vi "TCP Write Alive 2.vi"(0 "remote port or service name":u16=6341, 1 "MultiCast Port":u16=58432, 3 "Stopqueue":refnum<queue>, 5 "address":string="localhost", 7 "Stop":bool, 9 "Name":string="MyName 2", 11 "error in (no error)":errorcluster, 13 "MultiCast Address":string="234.5.6.7", 14 "stop":bool) -> (4 "Stop?":bool, 6 "PhysicalStop?":bool, 15 "error out":errorcluster)   [LabVIEW 2013]
uses:
  <vilib>/Utility/tcp.llb/UDP Multicast Read-Only Open.vi
panel:
  out "stop 2":bool
  in  "OK":bool
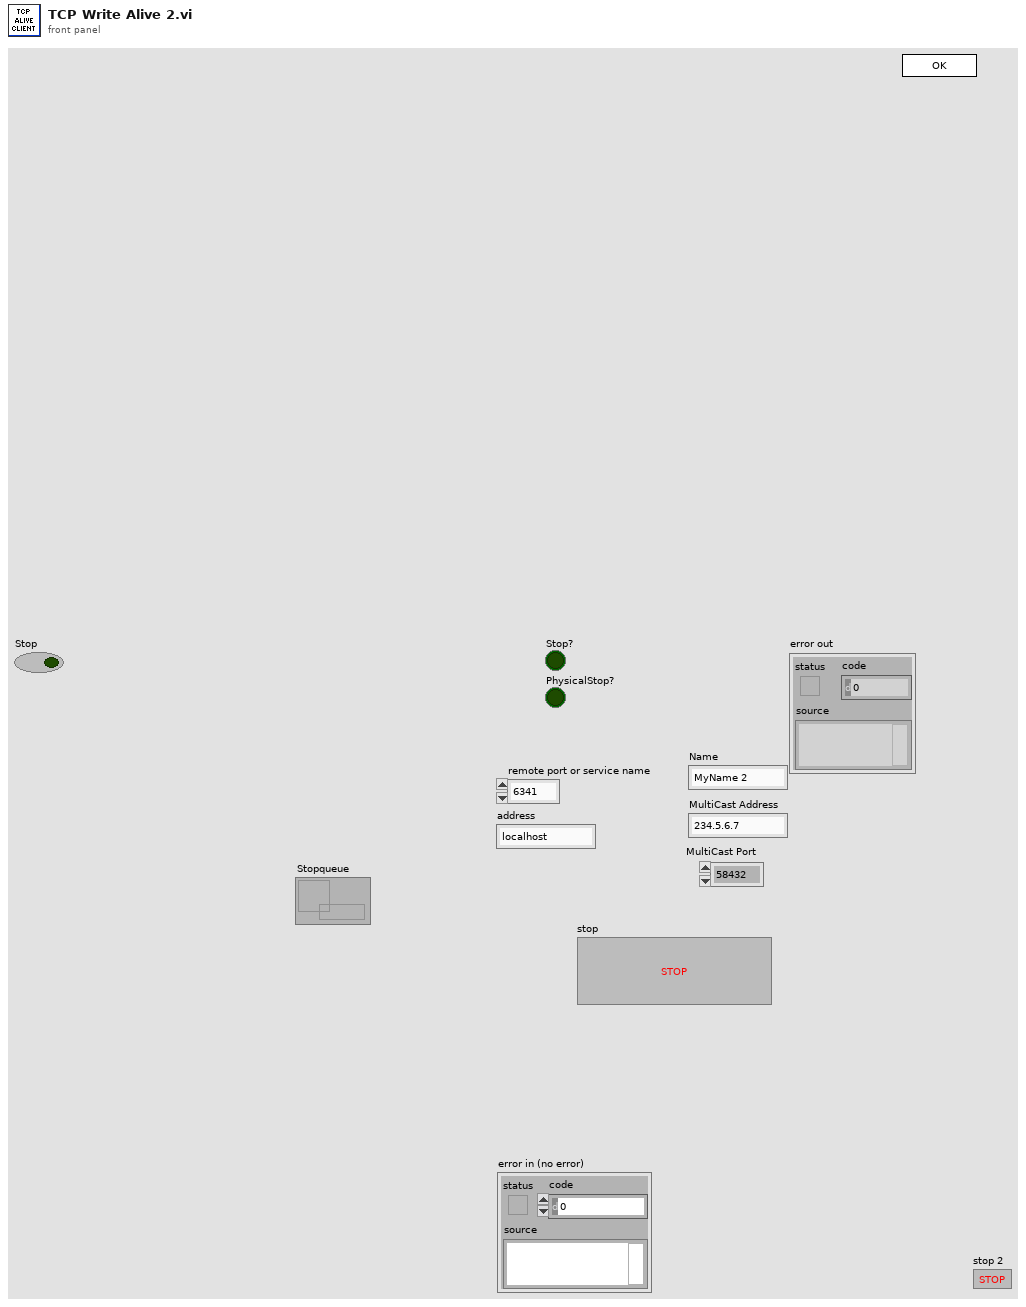
[diagram p1: front panel]
types:
  T1 = enum32{"invalid app kind", "Development System", "Run Time System", "Student Edition", "Embedded LabVIEW", "Evaluation", "Custom"}
  T2 = enum32{"Invalid", "Standard", "Closed", "Hidden", "Minimized", "Maximized"}
  T3 = cluster{"Core":cluster{"Current VI Reference":refnum<vi>, "Close Panel on Exit?":bool}, "PhysicalStop?":bool, "Alive String":string, "connection ID":refnum<k5>, "Address":string, "remote port or service name 2":u16, "Stop String":string}
  T4 = cluster{"Current VI Reference":refnum<vi>, "Close Panel on Exit?":bool}
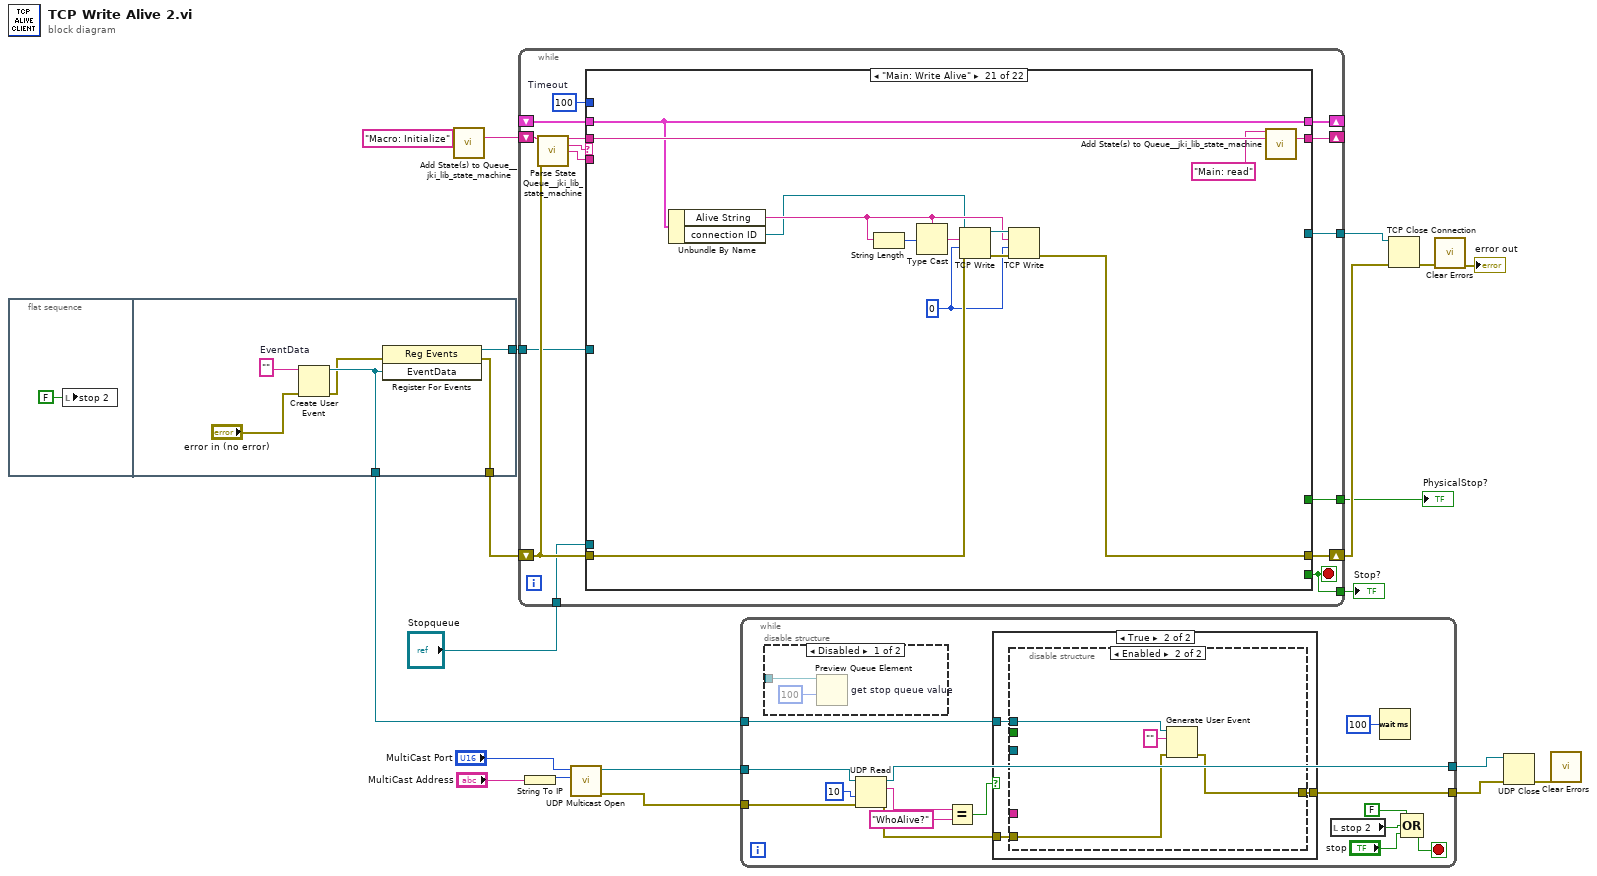
[diagram p0: block diagram]
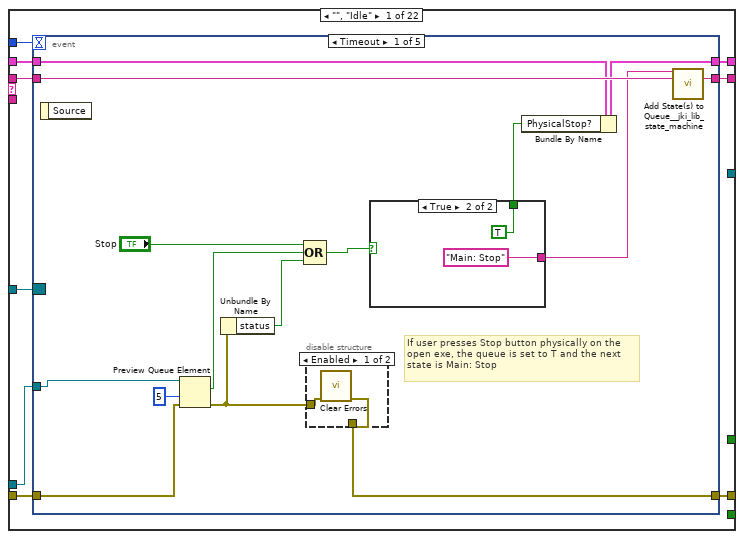
[diagram p2: hidden frame]
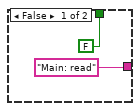
[diagram p4: hidden frame]
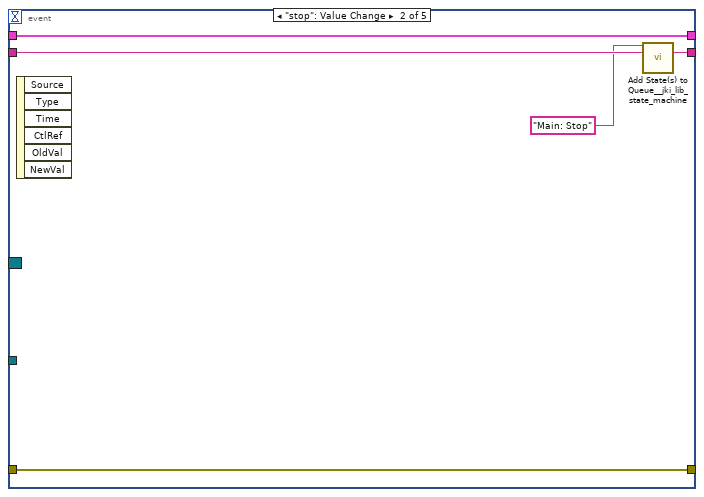
[diagram p5: hidden frame]
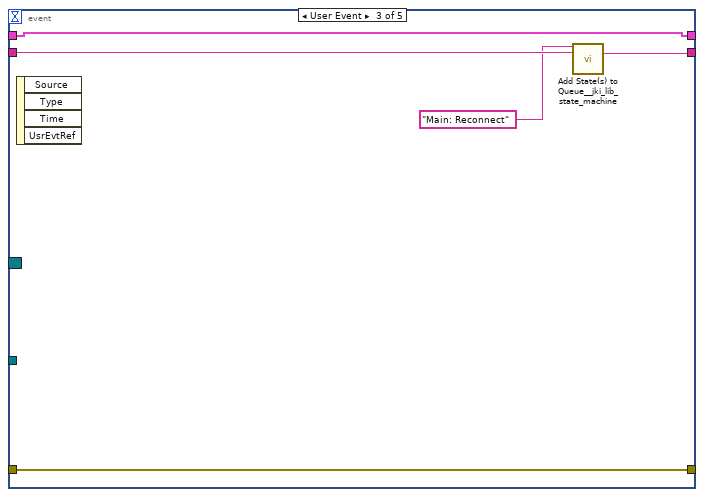
[diagram p6: hidden frame]
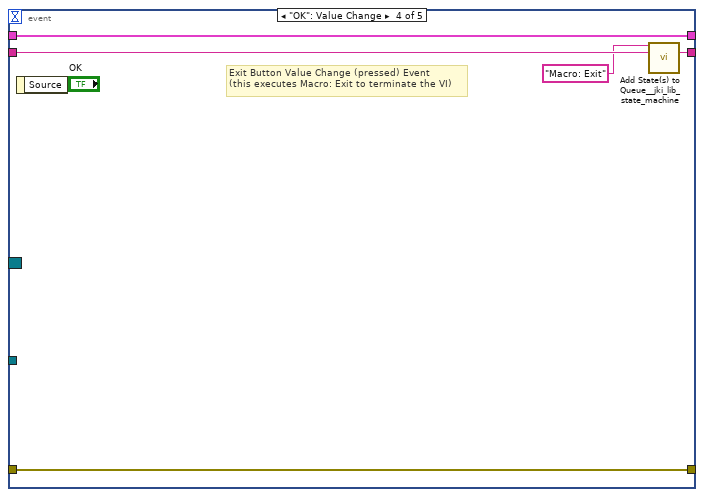
[diagram p7: hidden frame]
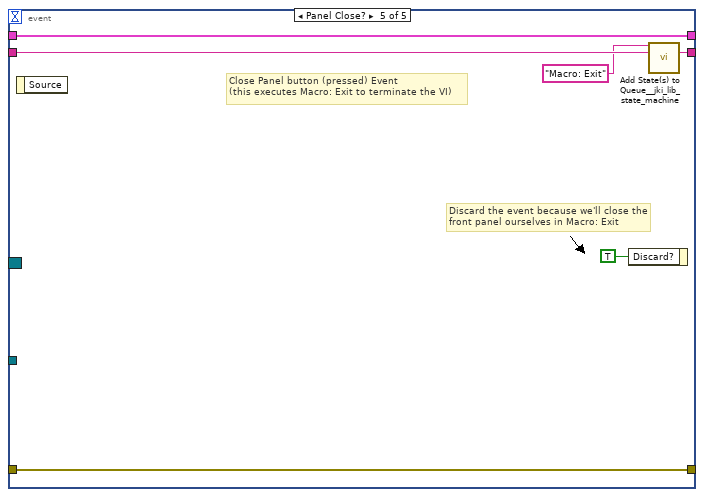
[diagram p8: hidden frame]
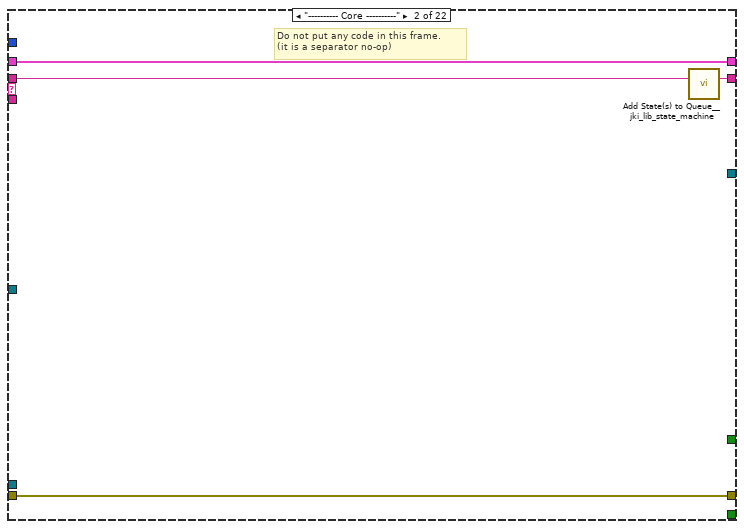
[diagram p9: hidden frame]
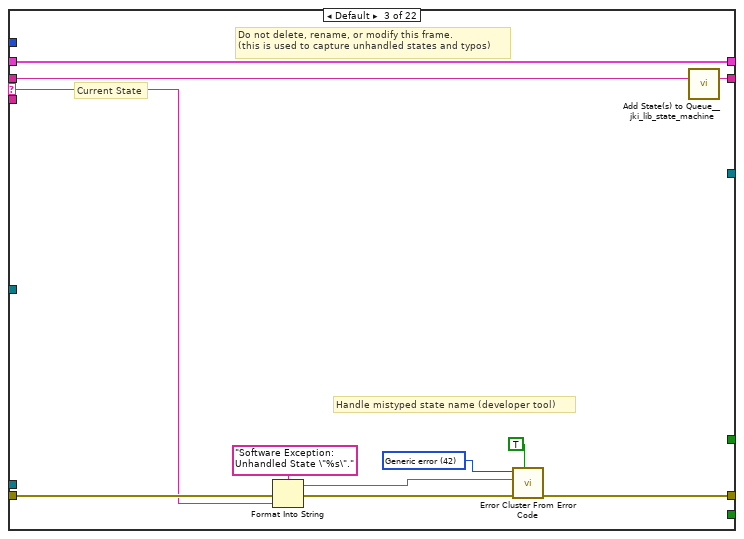
[diagram p10: hidden frame]
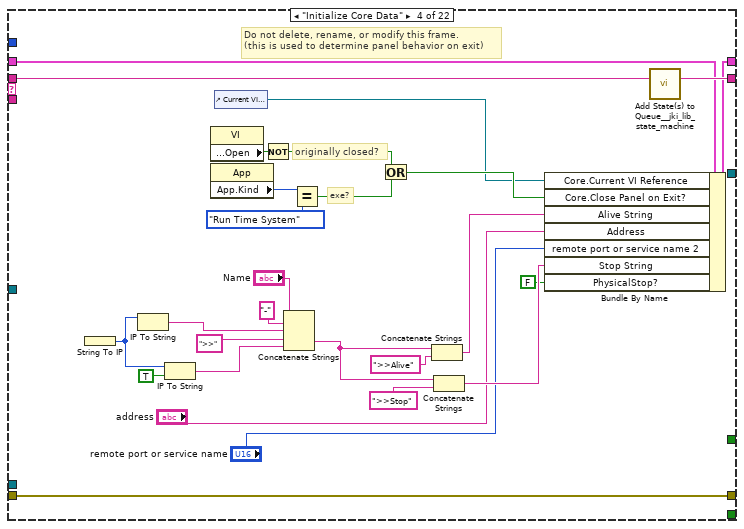
[diagram p11: hidden frame]
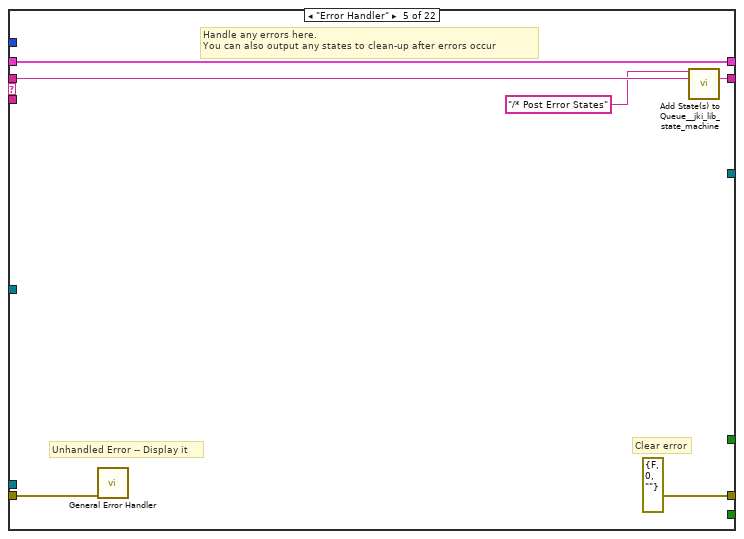
[diagram p12: hidden frame]
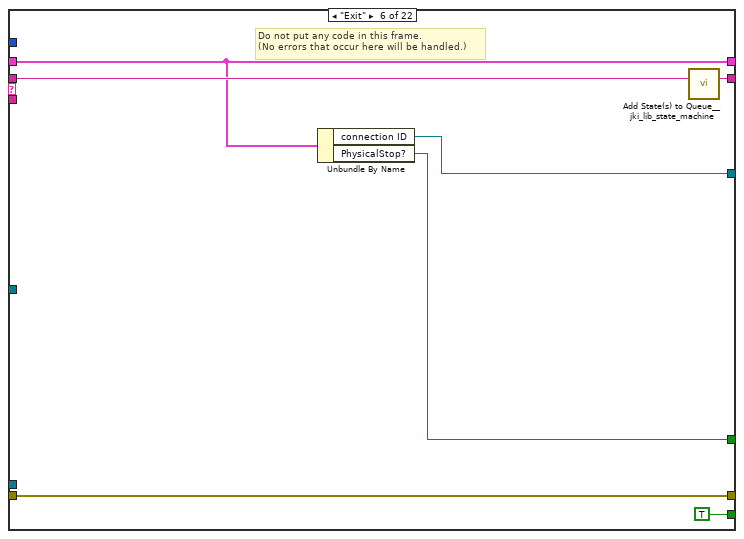
[diagram p13: hidden frame]
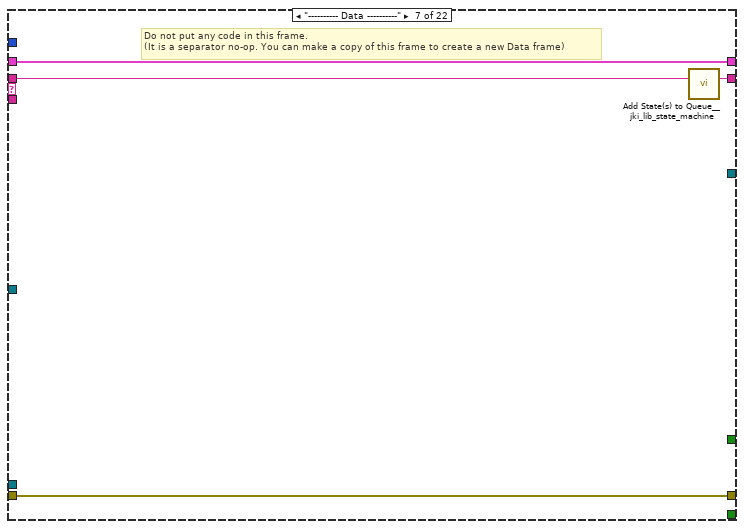
[diagram p14: hidden frame]
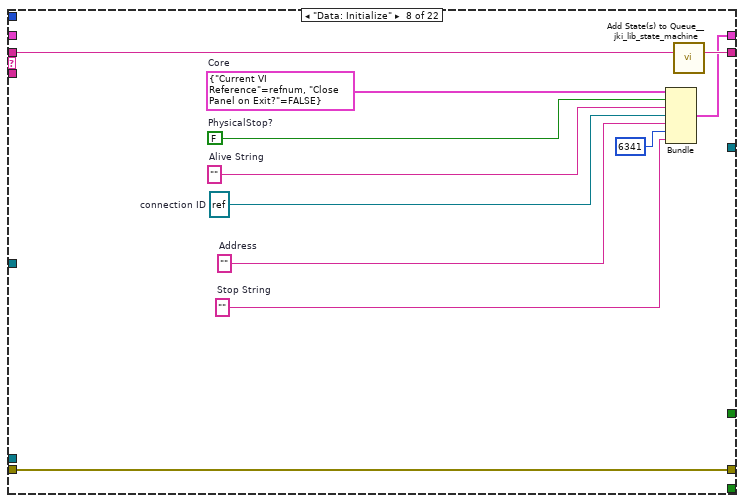
[diagram p15: hidden frame]
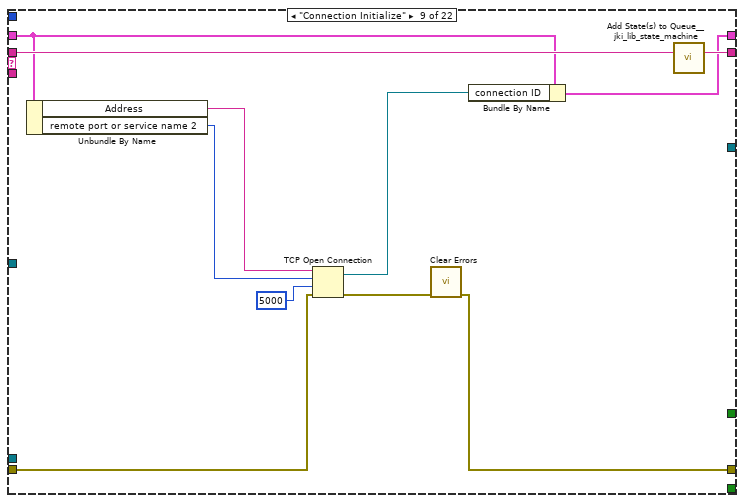
[diagram p16: hidden frame]
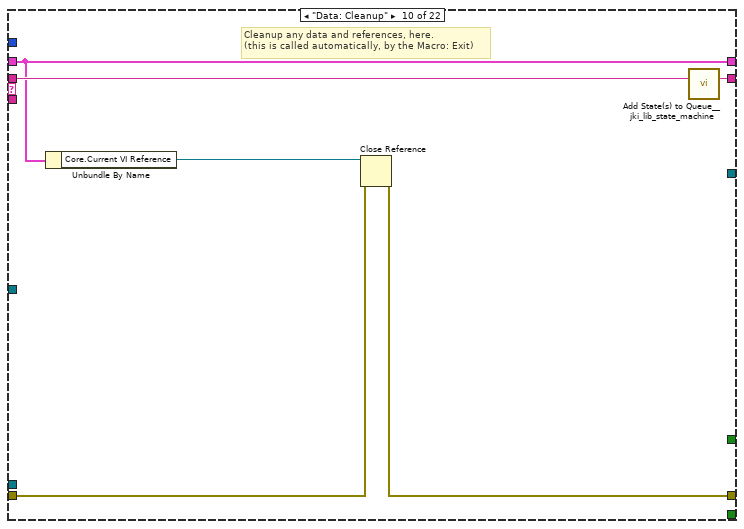
[diagram p17: hidden frame]
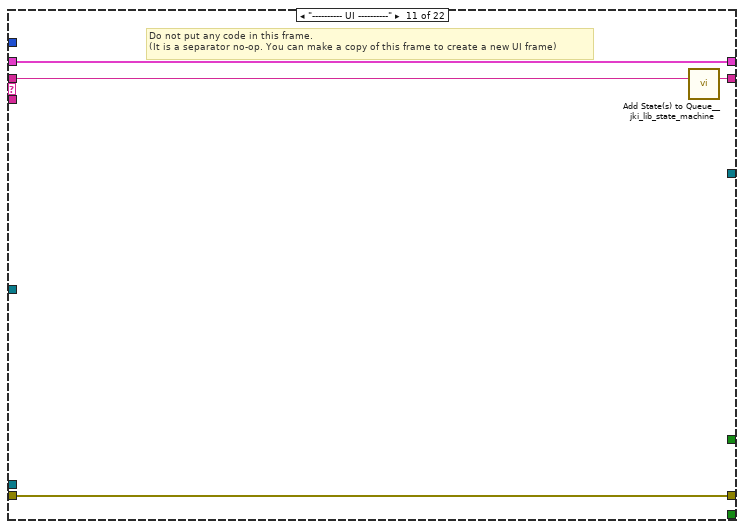
[diagram p18: hidden frame]
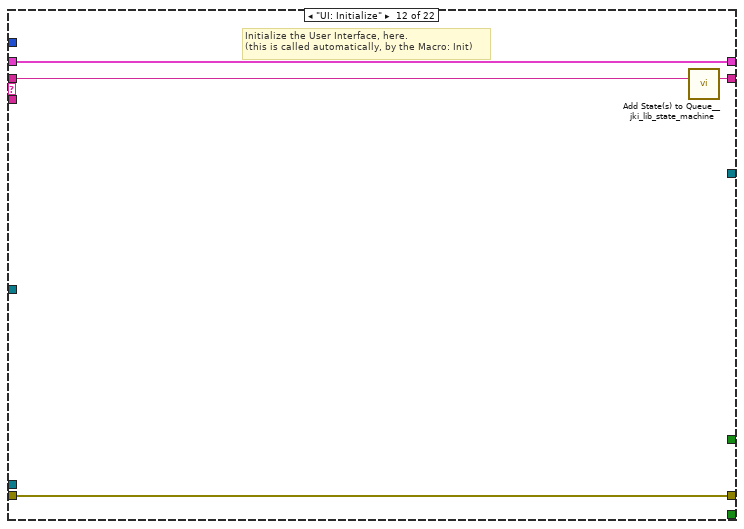
[diagram p19: hidden frame]
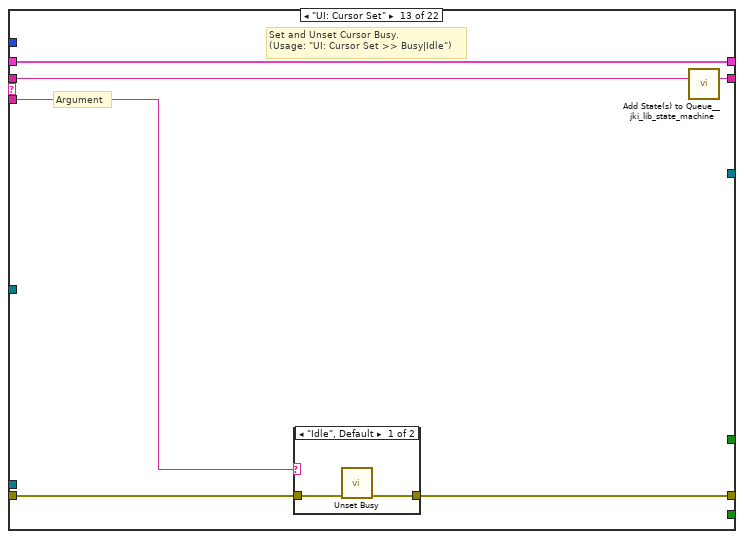
[diagram p20: hidden frame]
diagram:
  n1 = flat-sequence {
    tunnel: [w27] -> w11
    tunnel: [w25] -> w10
    tunnel: [w22] -> w9
    frame #0 {
      n2 = local write "stop 2"(FALSE ("stop 2")) -> ()
    }
    frame #1 {
      w26 = ""  # EventData
      n3 = Create User Event(user event datatype=w26, error in="error in (no error)") -> (user event=w25:refnum<user-event>, error out=w23:errorcluster)
      n4 = register-events(error in=w23, w25) -> (reference out=w27:refnum<event-registration>, error out=w22:errorcluster)  [unwired: 1 in]
    }
  }
  n5 = call <vilib>:"Add State(s) to Queue__jki_lib_state_machine.vi"("State(s) in (\"\")"="Macro: Initialize") -> ("States Out"=w13:string)  [unwired: 14 in]
  n6 = while {
    shift-right: [w36] -> _
    shift-left: _ -> [w35]
    shift-right: [w38] -> w6
    shift-left: w9 -> [w33]
    shift-right: [w37] -> _
    shift-left: w13 -> [w39]
    tunnel: w11 -> [w32]
    tunnel: [w31] -> w7
    tunnel: "Stopqueue" -> [w30]
    tunnel: [w29] -> w3
    tunnel: [w28] -> w1
    stop <- w29 stop-if-true
    w34 = 100  # Timeout
    n7 = call <vilib>:"Parse State Queue__jki_lib_state_machine.vi"("State Queue"=w39, "Error In (no error)"=w33) -> ("Remaining States"=w41:string, "Current State"=w42:string, "Arguments"=w40:string)  [unwired: 11 in]
    n8 = case shown="\"Main: Write Alive\"" w42 {
      selector: w42 -> [_ _ w99 _ _ _ _ _ _ _ _ _ _ _ _ _ _ _ _ _ _ _]
      tunnel: w41 -> [w51 w98 w103 w136 w142 w149 w153 w164 w175 w181 w185 w189 w195 w206 w232 w237 w247 w251 w266 w290 w322 w340]
      tunnel: w40 -> [_ _ _ _ _ _ _ _ _ _ _ _ w190 w200 _ _ _ _ _ _ _ _]
      tunnel: w35 -> [w49 w95 w101 w127 w139 w145 w150 _ w171 w176 w182 w187 w193 w202 w229 w234 w244 w248 w262 w273 w316 w334]
      tunnel: [w48 w96 w105 w133 errorcluster {"status"=FALSE, "code"=0, "source"=""} ("error out") w147 w151 w161 w166 w177 w183 w186 w191 w203 w230 w235 w245 w249 w254 w276 w310 w326] -> w38
      tunnel: w33 -> [w47 w96 w104 w133 w138 w147 w151 w161 w167 w178 w183 w186 w192 w204 w230 w235 w245 w249 w254 w277 w313 w331]
      tunnel: [w50 w97 w102 w135 w141 w148 w152 w163 w174 w180 w184 w188 w194 w205 w231 w236 w246 w250 w265 w289 w321 w339] -> w37
      tunnel: [_ _ _ _ _ TRUE _ _ _ _ _ _ _ _ _ _ _ _ _ _ _ _] -> w29
      tunnel: [w46 w95 w101 w134 w139 w145 w150 w162 w173 w176 w182 w187 w193 w202 w229 w234 w244 w248 w261 w272 w316 w334] -> w36
      tunnel: w34 -> [w45 _ _ _ _ _ _ _ _ _ _ _ _ _ _ _ _ _ _ _ _ _]
      tunnel: w32 -> [w44 _ _ _ _ _ _ _ _ _ _ _ _ _ _ _ _ _ _ _ _ _]
      tunnel: [_ _ _ _ _ w144 _ _ _ _ _ _ _ _ _ _ _ _ _ _ _ _] -> w31
      tunnel: w30 -> [w43 _ _ _ _ _ _ _ _ _ _ _ _ _ _ _ _ _ _ _ _ w325]
      tunnel: [_ _ _ _ _ w143 _ _ _ _ _ _ _ _ _ _ _ _ _ _ _ _] -> w28
      frame "", "Idle" {
        n9 = event shown="[0] Timeout" {
          selector: w44 -> [_ _ _ _ _]
          dyn-events: _ -> [_ _ _ _ _]
          timeout: w45 -> [_ _ _ _ _]
          tunnel: w51 -> [w66 w77 w82 w88 w94]
          tunnel: [w65 w78 w83 w87 w93] -> w50
          tunnel: w49 -> [w61 w76 w80 w85 w91]
          tunnel: [w57 w74 w79 w86 w92] -> w48
          tunnel: w47 -> [w58 w74 w79 w86 w92]
          tunnel: [w60 w76 w80 w85 w91] -> w46
          tunnel: w43 -> [w63 _ _ _ _]
          event Timeout {
            # "If user presses Stop button physically on the\nopen exe, the queue is set to T and the next\nstate is Main: Stop"
            n10 = event-data() -> ()  [unwired: 1 in, 1 out]
            n11 = Preview Queue Element ("get stop queue value")(queue=w63, timeout in ms (-1)=5, error in (no error)=w58) -> (element=w55:bool, error out=w53:errorcluster)  [unwired: 2 out]
            n12 = Unbundle By Name(w53) -> ("status"=w52:bool)
            n13 = Compound Arithmetic op=OR("Stop", w55, w52) -> (w54:bool)
            n14 = disable-structure shown="Enabled" {
              disable-tunnel: w53 -> [w68 w69]
              disable-tunnel: [w67 w69] -> w57
              frame Enabled {
                n15 = call <vilib>:"Clear Errors.vi"("error in (no error)"=w68) -> ("error out"=w67:errorcluster)  [unwired: 6 in]
              }
              frame Disabled {
              }
            }
            n16 = case shown="True" w54 {
              tunnel: ["Main: read" ("State(s) in Front (\"\")") "Main: Stop" ("State(s) in Front (\"\")")] -> w62
              tunnel: [FALSE TRUE] -> w59
              frame False {
              }
              frame True {
              }
            }
            n17 = Bundle By Name(cluster=w61, "PhysicalStop?"=w59) -> (w60:T3)
            n18 = call <vilib>:"Add State(s) to Queue__jki_lib_state_machine.vi"("State(s) in Front (\"\")"=w62, "State(s) in (\"\")"=w66) -> ("States Out"=w65:string)  [unwired: 13 in]
          }
          event "stop": Value Change {
            n19 = event-data() -> ()  [unwired: 1 in, 6 out]
            n20 = call <vilib>:"Add State(s) to Queue__jki_lib_state_machine.vi"("State(s) in Front (\"\")"="Main: Stop" ("State(s) in Front (\"\")"), "State(s) in (\"\")"=w77) -> ("States Out"=w78:string)  [unwired: 13 in]
          }
          event User Event {
            n21 = event-data() -> ()  [unwired: 1 in, 4 out]
            n22 = call <vilib>:"Add State(s) to Queue__jki_lib_state_machine.vi"("State(s) in Front (\"\")"="Main: Reconnect" ("State(s) in Front (\"\")"), "State(s) in (\"\")"=w82) -> ("States Out"=w83:string)  [unwired: 13 in]
          }
          event "OK": Value Change {
            # "Exit Button Value Change (pressed) Event\n(this executes Macro: Exit to terminate the VI)"
            n23 = event-data() -> ()  [unwired: 1 in, 1 out]
            n24 = call <vilib>:"Add State(s) to Queue__jki_lib_state_machine.vi"("State(s) in Front (\"\")"="Macro: Exit", "State(s) in (\"\")"=w88) -> ("States Out"=w87:string)  [unwired: 13 in]
          }
          event Panel Close? {
            # "Discard the event because we'll close the front panel ourselves in Macro: Exit"
            # "Close Panel button (pressed) Event\n(this executes Macro: Exit to terminate the VI)"
            n25 = event-data() -> ()  [unwired: 1 in, 1 out]
            n26 = event-data("Discard?"=TRUE) -> ()  [unwired: 1 in, 1 out]
            n27 = call <vilib>:"Add State(s) to Queue__jki_lib_state_machine.vi"("State(s) in Front (\"\")"="Macro: Exit", "State(s) in (\"\")"=w94) -> ("States Out"=w93:string)  [unwired: 13 in]
          }
        }
      }
      frame "---------- Core ----------" {
        # "Do not put any code in this frame.\n(it is a separator no-op)"
        n28 = call <vilib>:"Add State(s) to Queue__jki_lib_state_machine.vi"("State(s) in (\"\")"=w98) -> ("States Out"=w97:string)  [unwired: 14 in]
      }
      frame Default {
        w108 = 42 items=["No error", "Argument error", "Memory is full", "Out of zone", "End of file", "File already open", "Generic file I/O error", "File not found", "File permission error", "Disk is full", "Duplicate path", "Too many files open", "System feature not enabled", "Resource file not found", "Cannot add resource", "Resource not found", "Image not found", "Image memory error", "Pen does not exist", "Config type invalid", "Config token not found", "Config parse error", "Config memory error", "Bad external code format", "Bad external code offset", "External code not present", "Null window", "Destroy window error", "Null menu", "Print aborted", "Bad print record", "Print driver error", "Windows error during printing", "Memory error during printing", "Print dialog error", "Generic print error", "Invalid device refnum", "Device not found", "Device parameter error", "Device unit error", "Cannot open device", "Device call aborted", "Generic error", "Cancelled by user", "Object ID too low", "Object ID too high", "Object not in heap", "Unknown heap", "Unknown object (invalid DefProc)", "Unknown object (DefProc not in table)", "Message out of range", "Invalid (null) method", "Unknown message", "Manager call not supported", "Bad address", "Network operation in progress", "Network operation timed out", "Connection is busy", "Network attribute not supported", "Network error", "Address in use", "System out of memory", "Connection aborted", "Connection refused", "Not connected", "Already connected", "Connection closed", "Initialization error (interapplication manager)", "Bad occurrence", "Wait on unbound occurrence handler", "Occurrence queue overflow", "Datalog type conflict", "Unused", "Unrecognized type (interapplication manager)", "Memory corrupt", "Failed to make temporary DLL", "Old CIN version", "Drag socket not found", "Failed to load drop-object", "Failed to register OLE object", "Failed to release OLE object", "Format specifier type mismatch", "Unknown format specifier", "Too few format specifiers", "Too many format specifiers", "Scan failed", "Newer CIN version", "Error converting to variant", "Runtime menu error", "Password tampered", "Variant attribute not found", "Incompatible variant data type", "Event data is not available", "Event Store is not present", "Occurrence is not found", "Event Queue is not created", "Event info is not available", "Refnum passed is NULL", "Error retrieving Class GUID", "Error retrieving CoClass GUID", "Error retrieving TypeLib GUID.", "Bad built application magic bytes.", "Specific driver is different from the specific driver associated with the Logical Name.", "There is no session opened to the class driver.", "Max Error", "MAX - Error with config objects", "MAX - Error loading configuration", "MAX - Group not supported"]
        # "Current State"
        # "Do not delete, rename, or modify this frame.\n(this is used to capture unhandled states and typos)"
        # "Handle mistyped state name (developer tool)"
        n29 = Format Into String(format string="Software Exception: Unhandled State \"%s\"." ("message"), error in=w104, w99) -> (resulting string=w107:string, error out=w106:errorcluster)  [unwired: 1 in]
        n30 = call <vilib>:"Error Cluster From Error Code.vi"("show call chain? (False)"=TRUE, "error in (no error)"=w106, "error message (\"\")"=w107, "error code (0)"=w108) -> ("error out"=w105:errorcluster)  [unwired: 5 in]
        n31 = call <vilib>:"Add State(s) to Queue__jki_lib_state_machine.vi"("State(s) in (\"\")"=w103) -> ("States Out"=w102:string)  [unwired: 14 in]
      }
      frame "Initialize Core Data" {
        # "Do not delete, rename, or modify this frame.\n(this is used to determine panel behavior on exit)"
        # "originally closed?"
        # "exe?"
        n32 = String To IP() -> (0:w113:u32)  [unwired: 1 in]
        n33 = IP To String(2:w113) -> (0:w110:string)  [unwired: 1 in]
        n34 = IP To String(1:TRUE ("dot notation? (F)"), 2:w113) -> (0:w123:string)
        n35 = property class="VI"() -> ("Front Panel.Open"=w132:bool)  [unwired: 2 in, 2 out]
        n36 = property class="App"() -> ("App.Kind"=w131:T1)  [unwired: 2 in, 2 out]
        n37 = control-ref of="Current VI Reference"() -> (w125:refnum<vi>)
        n38 = Not(x=w132) -> (.not. x?=w129:bool)
        n39 = Concatenate Strings("Name", "-" ("string"), w110, ">>" ("string"), w123) -> (w120:string)
        n40 = Equal?(x=w131, y=T1."Run Time System" ("Application:Kind")) -> (x = y?=w128:bool)
        n41 = Or(x=w129, y=w128) -> (x .or. y?=w126:bool)
        n42 = Concatenate Strings(w120, ">>Alive" ("string")) -> (w121:string)
        n43 = Concatenate Strings(w120, ">>Stop" ("string")) -> (w118:string)
        n44 = Bundle By Name(cluster=w127, "Core.Current VI Reference"=w125, "Core.Close Panel on Exit?"=w126, "Alive String"=w121, "Address"="address", "remote port or service name 2"="remote port or service name", "Stop String"=w118, "PhysicalStop?"=FALSE) -> (w134:T3)
        n45 = call <vilib>:"Add State(s) to Queue__jki_lib_state_machine.vi"("State(s) in (\"\")"=w136) -> ("States Out"=w135:string)  [unwired: 14 in]
      }
      frame "Error Handler" {
        # "Unhandled Error -- Display it"
        # "Handle any errors here.\nYou can also output any states to clean-up after errors occur"
        # "Clear error"
        n46 = call <vilib>:"General Error Handler.vi"("error in (no error)"=w138) -> ()  [unwired: 10 in, 5 out]
        n47 = call <vilib>:"Add State(s) to Queue__jki_lib_state_machine.vi"("State(s) in Front (\"\")"="/* Post Error States", "State(s) in (\"\")"=w142) -> ("States Out"=w141:string)  [unwired: 13 in]
      }
      frame "Exit" {
        # "Do not put any code in this frame.\n(No errors that occur here will be handled.)"
        n48 = Unbundle By Name(w145) -> ("connection ID"=w144:refnum<k5>, "PhysicalStop?"=w143:bool)
        n49 = call <vilib>:"Add State(s) to Queue__jki_lib_state_machine.vi"("State(s) in (\"\")"=w149) -> ("States Out"=w148:string)  [unwired: 14 in]
      }
      frame "---------- Data ----------" {
        # "Do not put any code in this frame.\n(It is a separator no-op. You can make a copy of this frame to create a new Data frame)"
        n50 = call <vilib>:"Add State(s) to Queue__jki_lib_state_machine.vi"("State(s) in (\"\")"=w153) -> ("States Out"=w152:string)  [unwired: 14 in]
      }
      frame "Data: Initialize" {
        w154 = ""  # Stop String
        w156 = ""  # Address
        w157 = refnum<k5> refnum  # connection ID
        w158 = T4 {"Current VI Reference"=refnum, "Close Panel on Exit?"=FALSE}  # Core
        w160 = FALSE  # PhysicalStop?
        w159 = ""  # Alive String
        n51 = Bundle("Core"=w158, "PhysicalStop?"=w160, "Alive String"=w159, "connection ID"=w157, "Address"=w156, "remote port or service name 2"=u16 6341, "Stop String"=w154) -> (w162:T3)  [unwired: 1 in]
        n52 = call <vilib>:"Add State(s) to Queue__jki_lib_state_machine.vi"("State(s) in (\"\")"=w164) -> ("States Out"=w163:string)  [unwired: 14 in]
      }
      frame "Connection Initialize" {
        n53 = Unbundle By Name(w171) -> ("Address"=w170:string, "remote port or service name 2"=w169:u16)
        n54 = TCP Open Connection(address=w170, remote port or service name=w169, timeout ms (60000)=5000, error in (no error)=w167) -> (connection ID=w172:refnum<k5>, error out=w168:errorcluster)  [unwired: 1 in]
        n55 = call <vilib>:"Clear Errors.vi"("error in (no error)"=w168) -> ("error out"=w166:errorcluster)  [unwired: 6 in]
        n56 = Bundle By Name(cluster=w171, "connection ID"=w172) -> (w173:T3)
        n57 = call <vilib>:"Add State(s) to Queue__jki_lib_state_machine.vi"("State(s) in (\"\")"=w175) -> ("States Out"=w174:string)  [unwired: 14 in]
      }
      frame "Data: Cleanup" {
        # "Cleanup any data and references, here.\n(this is called automatically, by the Macro: Exit)"
        n58 = Unbundle By Name(w176) -> ("Core.Current VI Reference"=w179:refnum<vi>)
        n59 = Close Reference(reference=w179, error in (no error)=w178) -> (error out=w177:errorcluster)
        n60 = call <vilib>:"Add State(s) to Queue__jki_lib_state_machine.vi"("State(s) in (\"\")"=w181) -> ("States Out"=w180:string)  [unwired: 14 in]
      }
      frame "---------- UI ----------" {
        # "Do not put any code in this frame.\n(It is a separator no-op. You can make a copy of this frame to create a new UI frame)"
        n61 = call <vilib>:"Add State(s) to Queue__jki_lib_state_machine.vi"("State(s) in (\"\")"=w185) -> ("States Out"=w184:string)  [unwired: 14 in]
      }
      frame "UI: Initialize" {
        # "Initialize the User Interface, here.\n(this is called automatically, by the Macro: Init)"
        n62 = call <vilib>:"Add State(s) to Queue__jki_lib_state_machine.vi"("State(s) in (\"\")"=w189) -> ("States Out"=w188:string)  [unwired: 14 in]
      }
      frame "UI: Cursor Set" {
        # "Argument"
        # "Set and Unset Cursor Busy.\n(Usage: \"UI: Cursor Set >> Busy|Idle\")"
        n63 = case shown="\"Idle\", Default" w190 {
          tunnel: w192 -> [w197 w199]
          tunnel: [w196 w198] -> w191
          frame "Idle", Default {
            n64 = call <vilib>:"Unset Busy.vi"("error in (no error)"=w197) -> ("error out"=w196:errorcluster)  [unwired: 10 in]
          }
          frame "Busy" {
            n65 = call <vilib>:"Set Busy.vi"("error in (no error)"=w199) -> ("error out"=w198:errorcluster)  [unwired: 9 in, 1 out]
          }
        }
        n66 = call <vilib>:"Add State(s) to Queue__jki_lib_state_machine.vi"("State(s) in (\"\")"=w195) -> ("States Out"=w194:string)  [unwired: 14 in]
      }
      frame "UI: Front Panel State" {
        # "Argument"
        # "Set Front Panel Open or Closed\n(Usage: \"UI: Front Panel State >> Open|Close\")"
        n67 = Unbundle By Name(w202) -> ("Core.Current VI Reference"=w201:refnum<vi>)
        n68 = case shown="\"Open\", Default" w200 {
          tunnel: w204 -> [w210 w223]
          tunnel: [w212 w224] -> w203
          tunnel: w201 -> [w211 w221]
          frame "Open", Default {
            n69 = property class="VI"(reference=w211, error in=w210) -> (reference out=w208:refnum<vi>, error out=w209:errorcluster, "Front Panel.Open"=w207:bool)
            n70 = case shown="False" w207 {
              tunnel: [w215 w218] -> w212
              tunnel: w209 -> [w214 w218]
              tunnel: w208 -> [w213 _]
              frame False {
                n71 = invoke class="VI" method="FP.Open"(reference=w213, error in=w214, "Activate"=TRUE, "State"=T2."Standard") -> (error out=w215:errorcluster)  [unwired: 1 in, 4 out]
              }
              frame True {
              }
            }
          }
          frame "Close" {
            n72 = property class="VI"(reference=w221, error in=w223) -> (reference out=w220:refnum<vi>, error out=w222:errorcluster, "Front Panel.Open"=w219:bool)
            n73 = case shown="True" w219 {
              tunnel: [w225 w228] -> w224
              tunnel: w222 -> [w225 w227]
              tunnel: w220 -> [_ w226]
              frame False {
              }
              frame True {
                n74 = invoke class="VI" method="FP.Close"(reference=w226, error in=w227) -> (error out=w228:errorcluster)  [unwired: 1 in, 2 out]
              }
            }
          }
        }
        n75 = call <vilib>:"Add State(s) to Queue__jki_lib_state_machine.vi"("State(s) in (\"\")"=w206) -> ("States Out"=w205:string)  [unwired: 14 in]
      }
      frame "---------- Macro ----------" {
        # "Do not put any code in this frame.\n(It is a separator no-op. You can make a copy of this frame to create a new Macro frame)"
        n76 = call <vilib>:"Add State(s) to Queue__jki_lib_state_machine.vi"("State(s) in (\"\")"=w232) -> ("States Out"=w231:string)  [unwired: 14 in]
      }
      frame "Macro: Initialize" {
        # "Initialization Macro\n(This is called once, when the VI starts)"
        n77 = call <vilib>:"Add State(s) to Queue__jki_lib_state_machine.vi"("State(s) in Front (\"\")"="Data: Initialize\nInitialize Core Data", "State(s) in (\"\")"=w237) -> ("States Out"=w236:string)  [unwired: 13 in]
      }
      frame "Macro: Exit" {
        # "Exit Macro\n(This is called once, when the VI exits)"
        n78 = Unbundle By Name(w244) -> ("Core.Close Panel on Exit?"=w243:bool)
        n79 = Select(t="UI: Front Panel State >> Close", s=w243, f="") -> (s? t:f=w240:string)
        n80 = call <vilib>:"Add State(s) to Queue__jki_lib_state_machine.vi"("State(s) in (\"\")"=w240, "State(s) at Back (\"\")"="Data: Cleanup\nExit") -> ("States Out"=w238:string)  [unwired: 13 in]
        n81 = call <vilib>:"Add State(s) to Queue__jki_lib_state_machine.vi"("State(s) in Front (\"\")"=w238, "State(s) in (\"\")"=w247) -> ("States Out"=w246:string)  [unwired: 13 in]
      }
      frame "---------- New Category ----------" {
        # "Template Separator\n(You can make a copy of, or modify, this frame)"
        n82 = call <vilib>:"Add State(s) to Queue__jki_lib_state_machine.vi"("State(s) in (\"\")"=w251) -> ("States Out"=w250:string)  [unwired: 14 in]
      }
      frame "Main: Reconnect" {
        # "Your code here.\n(You can make a copy of, or modify, this frame)"
        n83 = Unbundle By Name(w262) -> ("Address"=w264:string, "remote port or service name 2"=w263:u16, "connection ID"=w255:refnum<k5>)
        n84 = TCP Close Connection(connection ID=w255, error in (no error)=w254) -> (error out=w256:errorcluster)  [unwired: 1 in, 1 out]
        n85 = call <vilib>:"Clear Errors.vi"("error in (no error)"=w256) -> ("error out"=w253:errorcluster)  [unwired: 6 in]
        n86 = TCP Open Connection(address=w264, remote port or service name=w263, timeout ms (60000)=1000, error in (no error)=w253) -> (connection ID=w260:refnum<k5>, error out=w257:errorcluster)  [unwired: 1 in]
        n87 = Bundle By Name(cluster=w262, "connection ID"=w260) -> (w261:T3)
        n88 = case shown="No Error" w257 {
          tunnel: w257 -> [w268 w271]
          tunnel: [w268 w271] -> w259
          tunnel: ["Main: Write Alive" ("State(s) in Front (\"\")") "Idle" ("State(s) in Front (\"\")")] -> w258
          frame No Error {
          }
          frame Error {
            n89 = Wait (ms)(milliseconds to wait=u32 100) -> ()  [unwired: 1 out]
          }
        }
        n90 = call <vilib>:"Clear Errors.vi"("error in (no error)"=w259) -> ()  [unwired: 6 in, 1 out]
        n91 = call <vilib>:"Add State(s) to Queue__jki_lib_state_machine.vi"("State(s) in (\"\")"=w266, "State(s) at Back (\"\")"=w258) -> ("States Out"=w265:string)  [unwired: 13 in]
      }
      frame "Main: read" {
        w287 = 500 ("timeout ms (25000)")
        w283 = 4
        # "Your code here.\n(You can make a copy of, or modify, this frame)"
        n92 = Unbundle By Name(w273) -> ("Stop String"=w279:string, "connection ID"=w281:refnum<k5>, "PhysicalStop?"=w274:bool)
        n93 = TCP Read(connection ID=w281, bytes to read=w283, error in (no error)=w277, 9:w287) -> (connection ID out=w285:refnum<k5>, data out=w282:string, error out=w286:errorcluster)  [unwired: 1 out]
        n94 = Type Cast(type=w283, x=w282) -> (*(type *) &x=w284:i32)
        n95 = TCP Read(connection ID=w285, bytes to read=w284, error in (no error)=w286, 9:w287) -> (data out=w280:string, error out=w278:errorcluster)  [unwired: 2 out]
        n96 = Unbundle By Name(w278) -> ("code"=w288:i32)
        n97 = case shown="1, 66" w288 {
          tunnel: w280 -> [w299 _]
          tunnel: w279 -> [w298 _]
          tunnel: w278 -> [w297 w308]
          tunnel: [w296 w307] -> w276
          tunnel: [w295 "Main: Reconnect" ("State(s) in Front (\"\")")] -> w275
          tunnel: w274 -> [w293 _]
          tunnel: w273 -> [w292 w306]
          tunnel: [w291 w306] -> w272
          frame 0, Default {
            n98 = call <vilib>:"Clear Errors.vi"("error in (no error)"=w297) -> ("error out"=w296:errorcluster)  [unwired: 6 in]
            n99 = Equal?(x=w298, y=w299) -> (x = y?=w294:bool)
            n100 = case shown="False" w294 {
              tunnel: ["Idle" ("State(s) in Front (\"\")") "Main: Stop" ("State(s) in Front (\"\")")] -> w295
              tunnel: w293 -> [_ _]
              tunnel: w292 -> [w300 w304]
              tunnel: [w300 w303] -> w291
              frame False {
              }
              frame True {
                n101 = Bundle By Name(cluster=w304, "PhysicalStop?"=FALSE) -> (w303:T3)
              }
            }
          }
          frame 1, 66 {
            n102 = call <vilib>:"Clear Errors.vi"("error in (no error)"=w308) -> ("error out"=w307:errorcluster)  [unwired: 6 in]
          }
        }
        n103 = call <vilib>:"Add State(s) to Queue__jki_lib_state_machine.vi"("State(s) in Front (\"\")"=w275, "State(s) in (\"\")"=w290) -> ("States Out"=w289:string)  [unwired: 13 in]
      }
      frame "Main: Write Alive" {
        w311 = 0 ("timeout ms (25000)")
        n104 = Unbundle By Name(w316) -> ("Alive String"=w315:string, "connection ID"=w314:refnum<k5>)
        n105 = String Length(string=w315) -> (length=w319:i32)
        n106 = Type Cast(type=w315, x=w319) -> (*(type *) &x=w320:string)
        n107 = TCP Write(connection ID=w314, data in=w320, error in (no error)=w313, 9:w311) -> (connection ID out=w317:refnum<k5>, error out=w318:errorcluster)  [unwired: 1 out]
        n108 = TCP Write(connection ID=w317, data in=w315, error in (no error)=w318, 9:w311) -> (error out=w310:errorcluster)  [unwired: 2 out]
        n109 = call <vilib>:"Add State(s) to Queue__jki_lib_state_machine.vi"("State(s) in Front (\"\")"="Main: read" ("State(s) in Front (\"\")"), "State(s) in (\"\")"=w322) -> ("States Out"=w321:string)  [unwired: 13 in]
      }
      frame "Main: Stop" {
        w327 = 0 ("timeout ms (25000)")
        n110 = Unbundle By Name(w334) -> ("Stop String"=w333:string, "connection ID"=w332:refnum<k5>)
        n111 = String Length(string=w333) -> (length=w337:i32)
        n112 = Type Cast(type=w333, x=w337) -> (*(type *) &x=w338:string)
        n113 = TCP Write(connection ID=w332, data in=w338, error in (no error)=w331, 9:w327) -> (connection ID out=w335:refnum<k5>, error out=w336:errorcluster)  [unwired: 1 out]
        n114 = TCP Write(connection ID=w335, data in=w333, error in (no error)=w336, 9:w327) -> (error out=w330:errorcluster)  [unwired: 2 out]
        n115 = call <vilib>:"Clear Errors.vi"("error in (no error)"=w330) -> ("error out"=w326:errorcluster)  [unwired: 6 in]
        n116 = Lossy Enqueue Element(queue=w325, element=TRUE, error in (no error)=w326) -> (error out=w323:errorcluster)  [unwired: 3 out]
        n117 = call <vilib>:"Clear Errors.vi"("error in (no error)"=w323) -> ()  [unwired: 6 in, 1 out]
        n118 = call <vilib>:"Add State(s) to Queue__jki_lib_state_machine.vi"("State(s) in Front (\"\")"="Macro: Exit" ("State(s) in Front (\"\")"), "State(s) in (\"\")"=w340) -> ("States Out"=w339:string)  [unwired: 13 in]
        "stop 2" <- TRUE ("stop 2")
      }
    }
  }
  "Stop?" <- w3
  "PhysicalStop?" <- w1
  n119 = String To IP(1:"MultiCast Address") -> (0:w15:u32)
  n120 = call-poly <vilib>:"UDP Multicast Open.vi"("multicast addr"=w15, "port"="MultiCast Port") -> ("error out"=w19:errorcluster, "connection ID"=w18:refnum<k16>)  [unwired: 7 in, 1 out]
  n121 = while {
    tunnel: w19 -> [w354]
    tunnel: w18 -> [w353]
    tunnel: [w350] -> w17
    tunnel: [w348] -> w16
    tunnel: w10 -> [w346]
    stop <- w342 stop-if-true
    n122 = disable-structure shown="Disabled" {
      disable-tunnel: _ -> [w356 _]
      frame Disabled {
        n123 = Preview Queue Element "get stop queue value"(queue=w356, timeout in ms (-1)=100) -> ()  [unwired: 1 in, 4 out]
      }
      frame Enabled {
      }
    }
    n124 = UDP Read(connection ID=w353, timeout ms (25000)=10, 8:w354) -> (data out=w352:string, error out=w349:errorcluster, 3:w350:refnum<k16>)  [unwired: 1 in, 2 out]
    n125 = Equal?(x=w352, y="WhoAlive?") -> (x = y?=w347:bool)
    n126 = case shown="True" w347 {
      tunnel: w349 -> [w358 w361]
      tunnel: [w358 w360] -> w348
      tunnel: w346 -> [_ w359]
      frame False {
      }
      frame True {
        n127 = disable-structure shown="Enabled" {
          disable-tunnel: _ -> [w368 _]
          disable-tunnel: w361 -> [w367 w379]
          disable-tunnel: [w365 w378] -> w360
          disable-tunnel: _ -> [w364 _]
          disable-tunnel: _ -> [w362 _]
          disable-tunnel: w359 -> [_ w381]
          frame Disabled {
            n128 = case shown="True" w364 {
              tunnel: [w373 w374] -> w363
              tunnel: w362 -> [w373 _]
              frame False {
              }
              frame True {
                n129 = property on="remote port or service name" class="DigNum (strict)"() -> (error out=w376:errorcluster, "Value"=w375:u16)  [unwired: 2 in, 1 out]
                n130 = property on="address" class="Str"() -> ("Value"=w377:string)  [unwired: 2 in, 2 out]
                n131 = TCP Open Connection(address=w377, remote port or service name=w375, error in (no error)=w376) -> (connection ID=w374:refnum<k5>)  [unwired: 2 in, 1 out]
              }
            }
            n132 = String Length(string=w368) -> (length=w371:i32)
            n133 = Type Cast(type=w368, x=w371) -> (*(type *) &x=w372:string)
            n134 = TCP Write(connection ID=w363, data in=w372, error in (no error)=w367) -> (connection ID out=w370:refnum<k5>, error out=w366:errorcluster)  [unwired: 1 in, 1 out]
            n135 = TCP Write(connection ID=w370, data in=w368, error in (no error)=w366, 9:0 ("timeout ms (25000)")) -> (error out=w365:errorcluster)  [unwired: 2 out]
          }
          frame Enabled {
            n136 = Generate User Event(user event=w381, event data cluster="" ("event data"), error in=w379) -> (error out=w378:errorcluster)  [unwired: 1 in, 1 out]
          }
        }
      }
    }
    n137 = local read "stop 2"() -> (w343:bool)
    n138 = Wait (ms)(milliseconds to wait=u32 100) -> ()  [unwired: 1 out]
    n139 = Compound Arithmetic op=OR(FALSE ("value"), w343, "stop") -> (w342:bool)
  }
  n140 = TCP Close Connection(connection ID=w7, error in (no error)=w6) -> (error out=w5:errorcluster)  [unwired: 1 in, 1 out]
  n141 = call <vilib>:"Clear Errors.vi"("error in (no error)"=w5) -> ("error out"=→"error out":errorcluster)  [unwired: 6 in]
  n142 = UDP Close(connection ID=w17, 8:w16) -> (error out=w8:errorcluster)  [unwired: 1 out]
  n143 = call <vilib>:"Clear Errors.vi"("error in (no error)"=w8) -> ()  [unwired: 6 in, 1 out]
